vi "8bit try.vi"() -> ()   [LabVIEW 2020]
panel:
  out "SDI":u8[](array[numeric]) format="%.0x"
  out "error out":errorcluster
  out "Total Shifted Out":i32
  out "Actual Bitrate kHz":i32=1000
  in  "Rds per Sec":dbl=2000.0 max=2000000000.0
  out "SDO":u8[](array[numeric]) format="%.0x"
  in  "SCLK (kHz)":i32=2000 min=0
  out "Cheetah Handle":i32
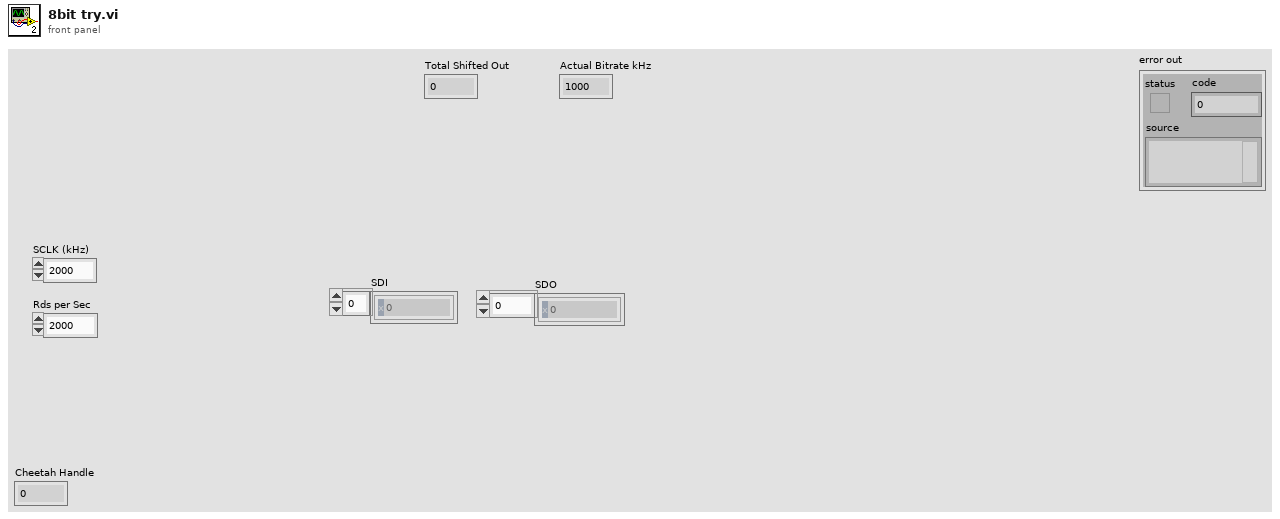
[diagram p1: front panel]
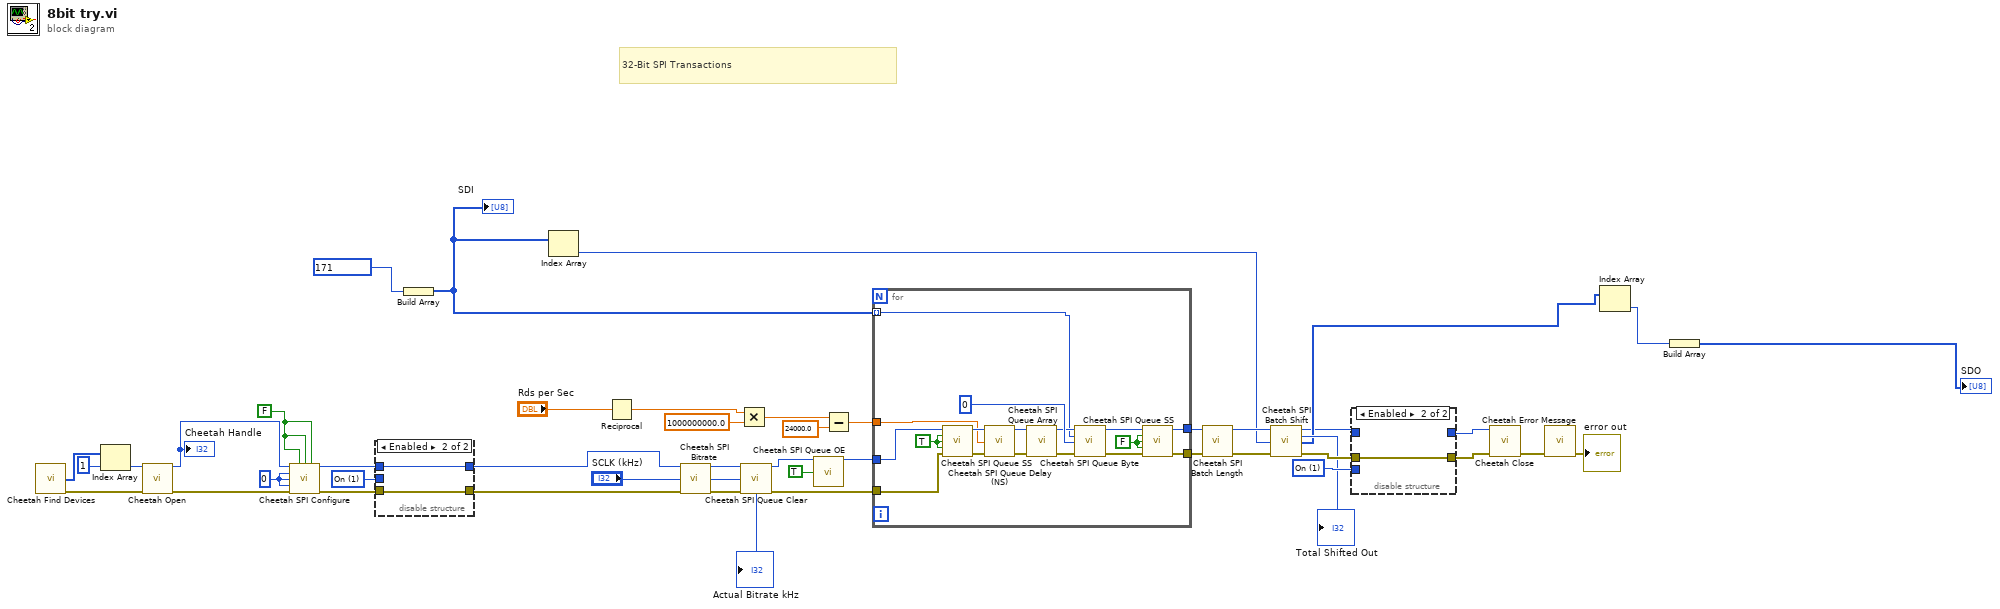
[diagram p0: block diagram]
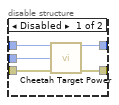
[diagram p2: hidden frame]
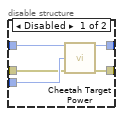
[diagram p3: hidden frame]
diagram:
  w25 = u16 1 items=["Off", "On", "Query"] ("Requested Configuration (2: Query)")
  w26 = u16 1 items=["Off", "On", "Query"] ("Requested Configuration (2: Query)")
  w41 = FALSE
  w43 = 0
  # "32-Bit SPI Transactions"
  n1 = call <instrlib>:"Cheetah Find Devices.vi"() -> ("Ports"=w44:u16[], "error out"=w40:errorcluster)  [unwired: 13 in, 1 out]
  n2 = Index Array(array=w44, index=1) -> (element=w32:u16)
  n3 = call <instrlib>:"Cheetah Open.vi"("Port Number (0)"=w32, "error in (no error)"=w40) -> ("Cheetah Handle"=w37:i32, "error out"=w39:errorcluster)  [unwired: 12 in]
  "Cheetah Handle" <- w37
  n4 = call <instrlib>:"Cheetah SPI Configure.vi"("Cheetah Handle"=w37, "SS0 Active High? (False)"=w41, "SS1 Active High? (False)"=w41, "SS2 Active High? (False)"=w41, "Polarity (0: Rising/Falling)"=w43, "Phase (0: Sample/Setup)"=w43, "Bitorder (0: MSB)"=w43, "error in (no error)"=w39) -> ("dup Cheetah Handle"=w36:i32, "error out"=w38:errorcluster)  [unwired: 6 in]
  n5 = disable-structure shown="Enabled" {
    disable-tunnel: w38 -> [w50 w51]
    disable-tunnel: w36 -> [w49 w52]
    disable-tunnel: [w48 w51] -> w35
    disable-tunnel: [w47 w52] -> w33
    disable-tunnel: w25 -> [w46 _]
    frame Disabled {
      n6 = call <instrlib>:"Cheetah Target Power.vi"("Cheetah Handle"=w49, "Requested Configuration (2: Query)"=w46, "error in (no error)"=w50) -> ("dup Cheetah Handle"=w47:i32, "error out"=w48:errorcluster)  [unwired: 10 in, 1 out]
    }
    frame Enabled {
    }
  }
  n7 = Build Array(u8 171 ("element")) -> (w6:u8[])
  "SDI" <- w6
  n8 = Index Array(array=w6) -> (element=w2:u8)  [unwired: 1 in]
  n9 = Reciprocal(x="Rds per Sec") -> (1/x=w11:dbl)
  n10 = call <instrlib>:"Cheetah SPI Bitrate.vi"("Cheetah Handle"=w33, "Requested Bitrate kHz (1000)"="SCLK (kHz)", "error in (no error)"=w35) -> ("dup Cheetah Handle"=w31:i32, "Actual Bitrate kHz"=→"Actual Bitrate kHz":i32, "error out"=w30:errorcluster)  [unwired: 10 in]
  n11 = Multiply(x=w11, y=1000000000.0) -> (x*y=w14:dbl)
  n12 = call <instrlib>:"Cheetah SPI Queue Clear.vi"("Cheetah Handle"=w31, "error in (no error)"=w30) -> ("dup Cheetah Handle"=w24:i32, "error out"=w42:errorcluster)  [unwired: 12 in]
  n13 = call <instrlib>:"Cheetah SPI Queue OE.vi"("Cheetah Handle"=w24, "Output Enable (on)"=TRUE) -> ("dup Cheetah Handle"=w23:i32)  [unwired: 12 in, 1 out]
  n14 = Subtract(x=w14, y=24000.0) -> (x-y=w12:dbl)
  n15 = for {
    tunnel: w42 -> [w59]
    tunnel: w23 -> [w60]
    tunnel: [w58] -> w21
    tunnel: [w57] -> w20
    tunnel: w12 -> [w55]
    tunnel: w6 -> [w53] mode=indexing
    w63 = FALSE
    w56 = TRUE
    n16 = call <instrlib>:"Cheetah SPI Queue SS.vi"("Cheetah Handle"=w60, "SS0 Assert? (True)"=w56, "SS1 Assert? (True)"=w56, "SS2 Assert? (True)"=w56, "error in (no error)"=w59) -> ("dup Cheetah Handle"=w69:i32, "error out"=w68:errorcluster)  [unwired: 9 in]
    n17 = call <instrlib>:"Cheetah SPI Queue Delay (NS).vi"("Cheetah Handle"=w69, "Delay NS (1000)"=w55, "error in (no error)"=w68) -> ("dup Cheetah Handle"=w67:i32, "error out"=w66:errorcluster)  [unwired: 10 in, 1 out]
    n18 = call <instrlib>:"Cheetah SPI Queue Array.vi"("Cheetah Handle"=w67, "error in (no error)"=w66) -> ("dup Cheetah Handle"=w54:i32, "error out"=w65:errorcluster)  [unwired: 12 in]
    n19 = call <instrlib>:"Cheetah SPI Queue Byte.vi"("Cheetah Handle"=w54, "Byte Count (1)"=w53, "Byte Value (0x00)"=0, "error in (no error)"=w65) -> ("dup Cheetah Handle"=w62:i32, "error out"=w61:errorcluster)  [unwired: 10 in]
    n20 = call <instrlib>:"Cheetah SPI Queue SS.vi"("Cheetah Handle"=w62, "SS0 Assert? (True)"=w63, "SS1 Assert? (True)"=w63, "SS2 Assert? (True)"=w63, "error in (no error)"=w61) -> ("dup Cheetah Handle"=w57:i32, "error out"=w58:errorcluster)  [unwired: 9 in]
  }
  n21 = call <instrlib>:"Cheetah SPI Batch Length.vi"("Cheetah Handle"=w20, "error in (no error)"=w21) -> ("dup Cheetah Handle"=w19:i32, "error out"=w18:errorcluster)  [unwired: 11 in, 1 out]
  n22 = call <instrlib>:"Cheetah SPI Batch Shift.vi"("Cheetah Handle"=w19, "Max Bytes to Retrieve (256)"=w2, "error in (no error)"=w18) -> ("dup Cheetah Handle"=w1:i32, "Total Shifted Out"=→"Total Shifted Out":i32, "Data In"=w5:u8[], "error out"=w17:errorcluster)  [unwired: 9 in]
  n23 = disable-structure shown="Enabled" {
    disable-tunnel: [w74 _] -> w29
    disable-tunnel: [w73 w75] -> w28
    disable-tunnel: w26 -> [w72 _]
    disable-tunnel: w1 -> [w71 _]
    disable-tunnel: w17 -> [w70 w75]
    frame Disabled {
      n24 = call <instrlib>:"Cheetah Target Power.vi"("Cheetah Handle"=w71, "Requested Configuration (2: Query)"=w72, "error in (no error)"=w70) -> ("dup Cheetah Handle"=w74:i32, "error out"=w73:errorcluster)  [unwired: 10 in, 1 out]
    }
    frame Enabled {
    }
  }
  n25 = call <instrlib>:"Cheetah Close.vi"("Cheetah Handle"=w29, "error in (no error)"=w28) -> ("error out"=w27:errorcluster)  [unwired: 12 in, 1 out]
  n26 = call <instrlib>:"Cheetah Error Message.vi"("error in (no error)"=w27) -> ("error out"=→"error out":errorcluster)  [unwired: 10 in, 4 out]
  n27 = Index Array(array=w5) -> (element=w4:u8)  [unwired: 1 in]
  n28 = Build Array(w4) -> (→"SDO":u8[])
